vi "Complex Combined System.vi"() -> ()   [LabVIEW 2017]
uses:
  <vilib>/userdefined/High Color/IMAQdx.ctl
  <vilib>/vision/driver/NI_Vision_Acquisition_Software.lvlib
  <vilib>/vision/NI_Vision_Development_Module.lvlib
panel:
  out "String":string
  in  "Send":bool
  out "error out":errorcluster
  out "size(s)":i32
  out "All Other IP Addresses":string
  out "Primary IP Address":string
  in  "Message":string
  in  "Subject":string
  in  "Recipients":string="chyslop@hotmail.co.uk, b8026896@my.shu.ac.uk,"
  in  "Noise IR Sensor 0 = no noise":dbl
  out "Output voltage":dbl
  in  "IR Object Distance":dbl(slide) min=0.0 max=100.0 step=1.0 scale=0.0..0.45
  out "Right Motor Speedometer (m/s)":dbl(knob) scale=-2.5..2.5
  out "Left Motor Speedometer (m/s)":dbl(knob) scale=-2.5..2.5
  in  "Noise Line sesnor 0 = no noise":dbl
  out "Right voltage more than 0?":bool
  out "Right Line sensor output voltage":dbl
  in  "Right Line Detector Sensor":dbl(slide) scale=0.0..5.0
  out "Left Voltage more than 0?":bool
  out "Left Line sensor output voltage":dbl
  in  "Left Line Detector Sensor":dbl(slide) scale=0.0..5.0
  out "Middle voltage more than 0?":bool
  out "Middle Line sensor output voltage":dbl
  in  "Middle Line Detector Sensor":dbl(slide) scale=0.0..5.0
  in  "% Power":dbl(slide) scale=0.0..100.0
  out "Direction":string
  out "Speedometer (m/s)":dbl(knob) scale=0.0..3.0
  out "error out 2":errorcluster
  out "Video Stream":T1(plugin-control)
  in  "stop":bool
  out "Found":bool
  out "Data":string
  out "error out 3":errorcluster
  out "error out 8":errorcluster
  out "error out 4":errorcluster
  in  "Barcode Types To Search":u32[](array[ring])=[6, 4] items=["Reserved", "Codabar", "Code 39", "Code 93", "Code 128", "EAN 8", "EAN 13", "Interleaved 2 of 5", "MSI", "UPCA", "Pharmacode", "RSS Limited"]
  out "error out 5":errorcluster
  in  "Select Vision System":string(combo)="None"
  in  "Session In":T2
  in  "Stop":bool
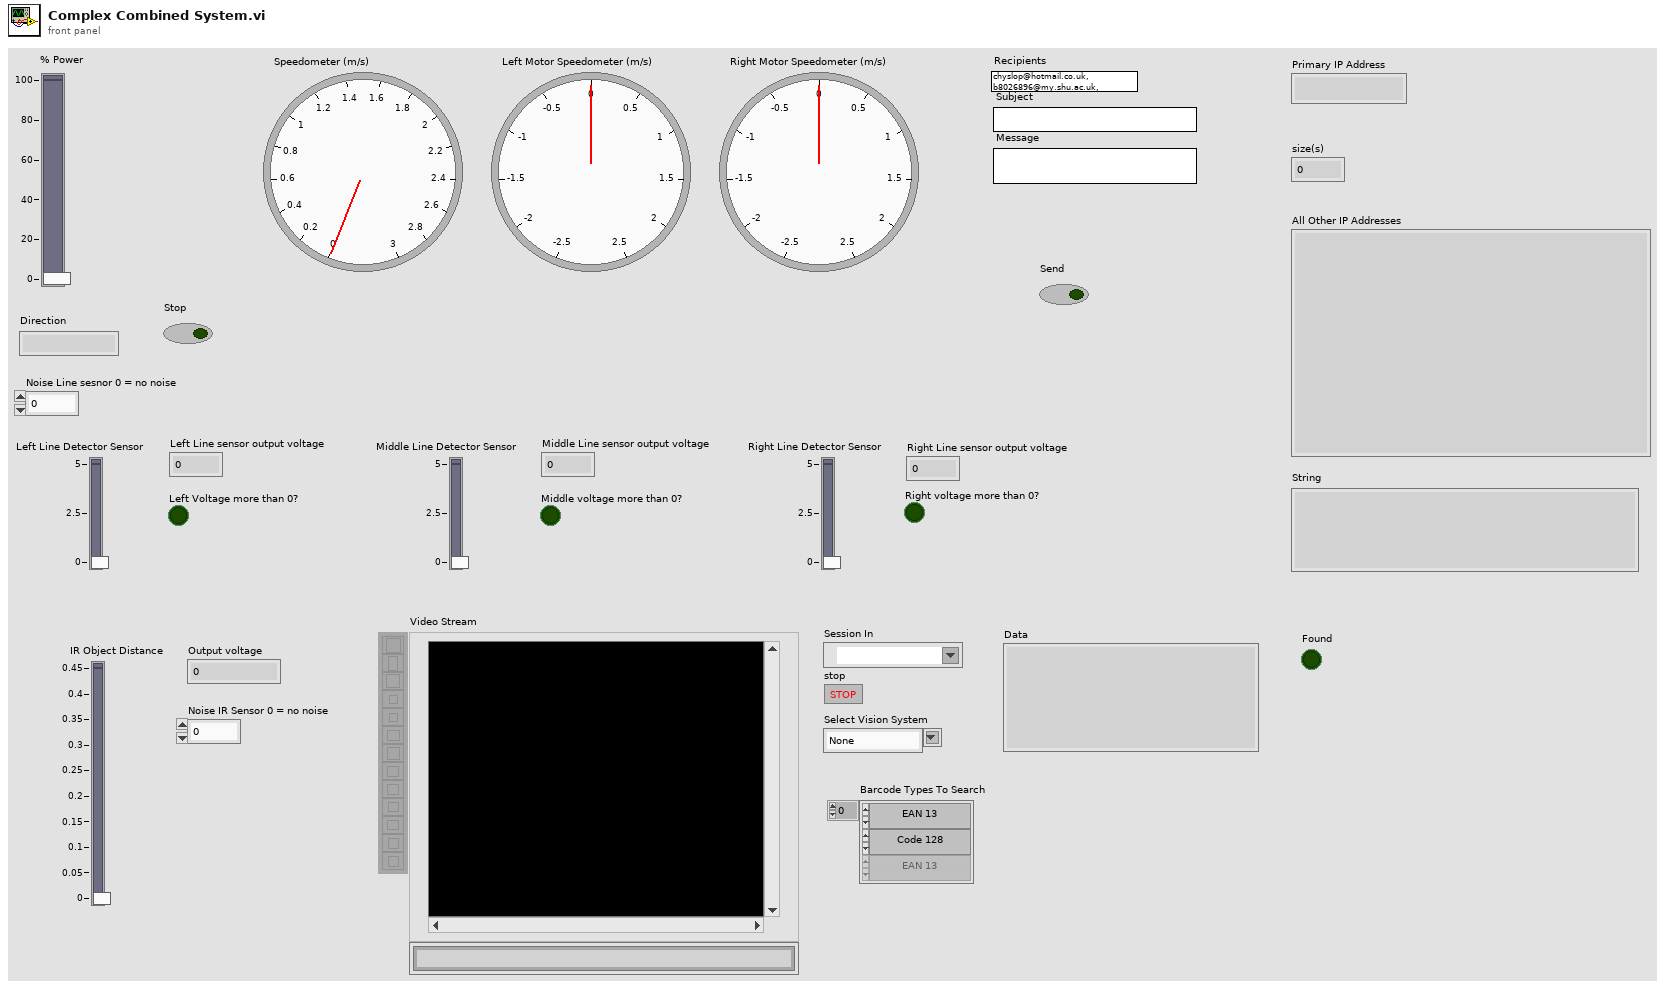
[diagram p1: front panel]
types:
  T1 = typedef "IMAQ Image.ctl" = refnum<image>
  T2 = typedef "IMAQdx.ctl" = refnum<k21>
  T3 = typedef "Image Type" = u32
  T4 = cluster{"Data":string, "Special Char 1":string, "Special Char 2":string, "Checksum(s)":string, "Barcode Type":u32, "Confidence Level":sgl, "Bounding Box":cluster{"x":sgl, "y":sgl}[]}[]
  T5 = cluster{"Data":string, "Special Char 1":string, "Special Char 2":string, "Checksum(s)":string, "Barcode Type":u32, "Confidence Level":sgl, "Bounding Box":cluster{"x":sgl, "y":sgl}[]}
  T6 = typedef "QR Code Report.ctl" = cluster{"Found?":bool, "Data":string, "Bounding Box":cluster{"x":sgl, "y":sgl}[], "Errors Corrected":u32, "Dimensions (Rows/Cols)":u32, "Version":u32, "QR Model":T7, "Stream Mode":T8, "Barcode Polarity":T9, "Mirrored?":bool, "Append Stream Position":u32, "Size of Append Stream":u32, "First EAN-128 ID":i32, "First Alternate Language ID":i32, "Append Stream ID":u32, "Minimum Edge Strength":u32, "Demodulation Mode":T10, "Cell Sample Size":T11, "Cell Filter Mode":T12}
  T7 = typedef "QR Code Model Type.ctl" = i32
  T8 = typedef "QR Code Stream Mode Type.ctl" = i32
  T9 = typedef "Data Matrix Polarity.ctl" = i32
  T10 = typedef "Demodulation Mode.ctl" = i32
  T11 = typedef "Cell Sample Size.ctl" = i32
  T12 = typedef "Cell Filter Mode.ctl" = i32
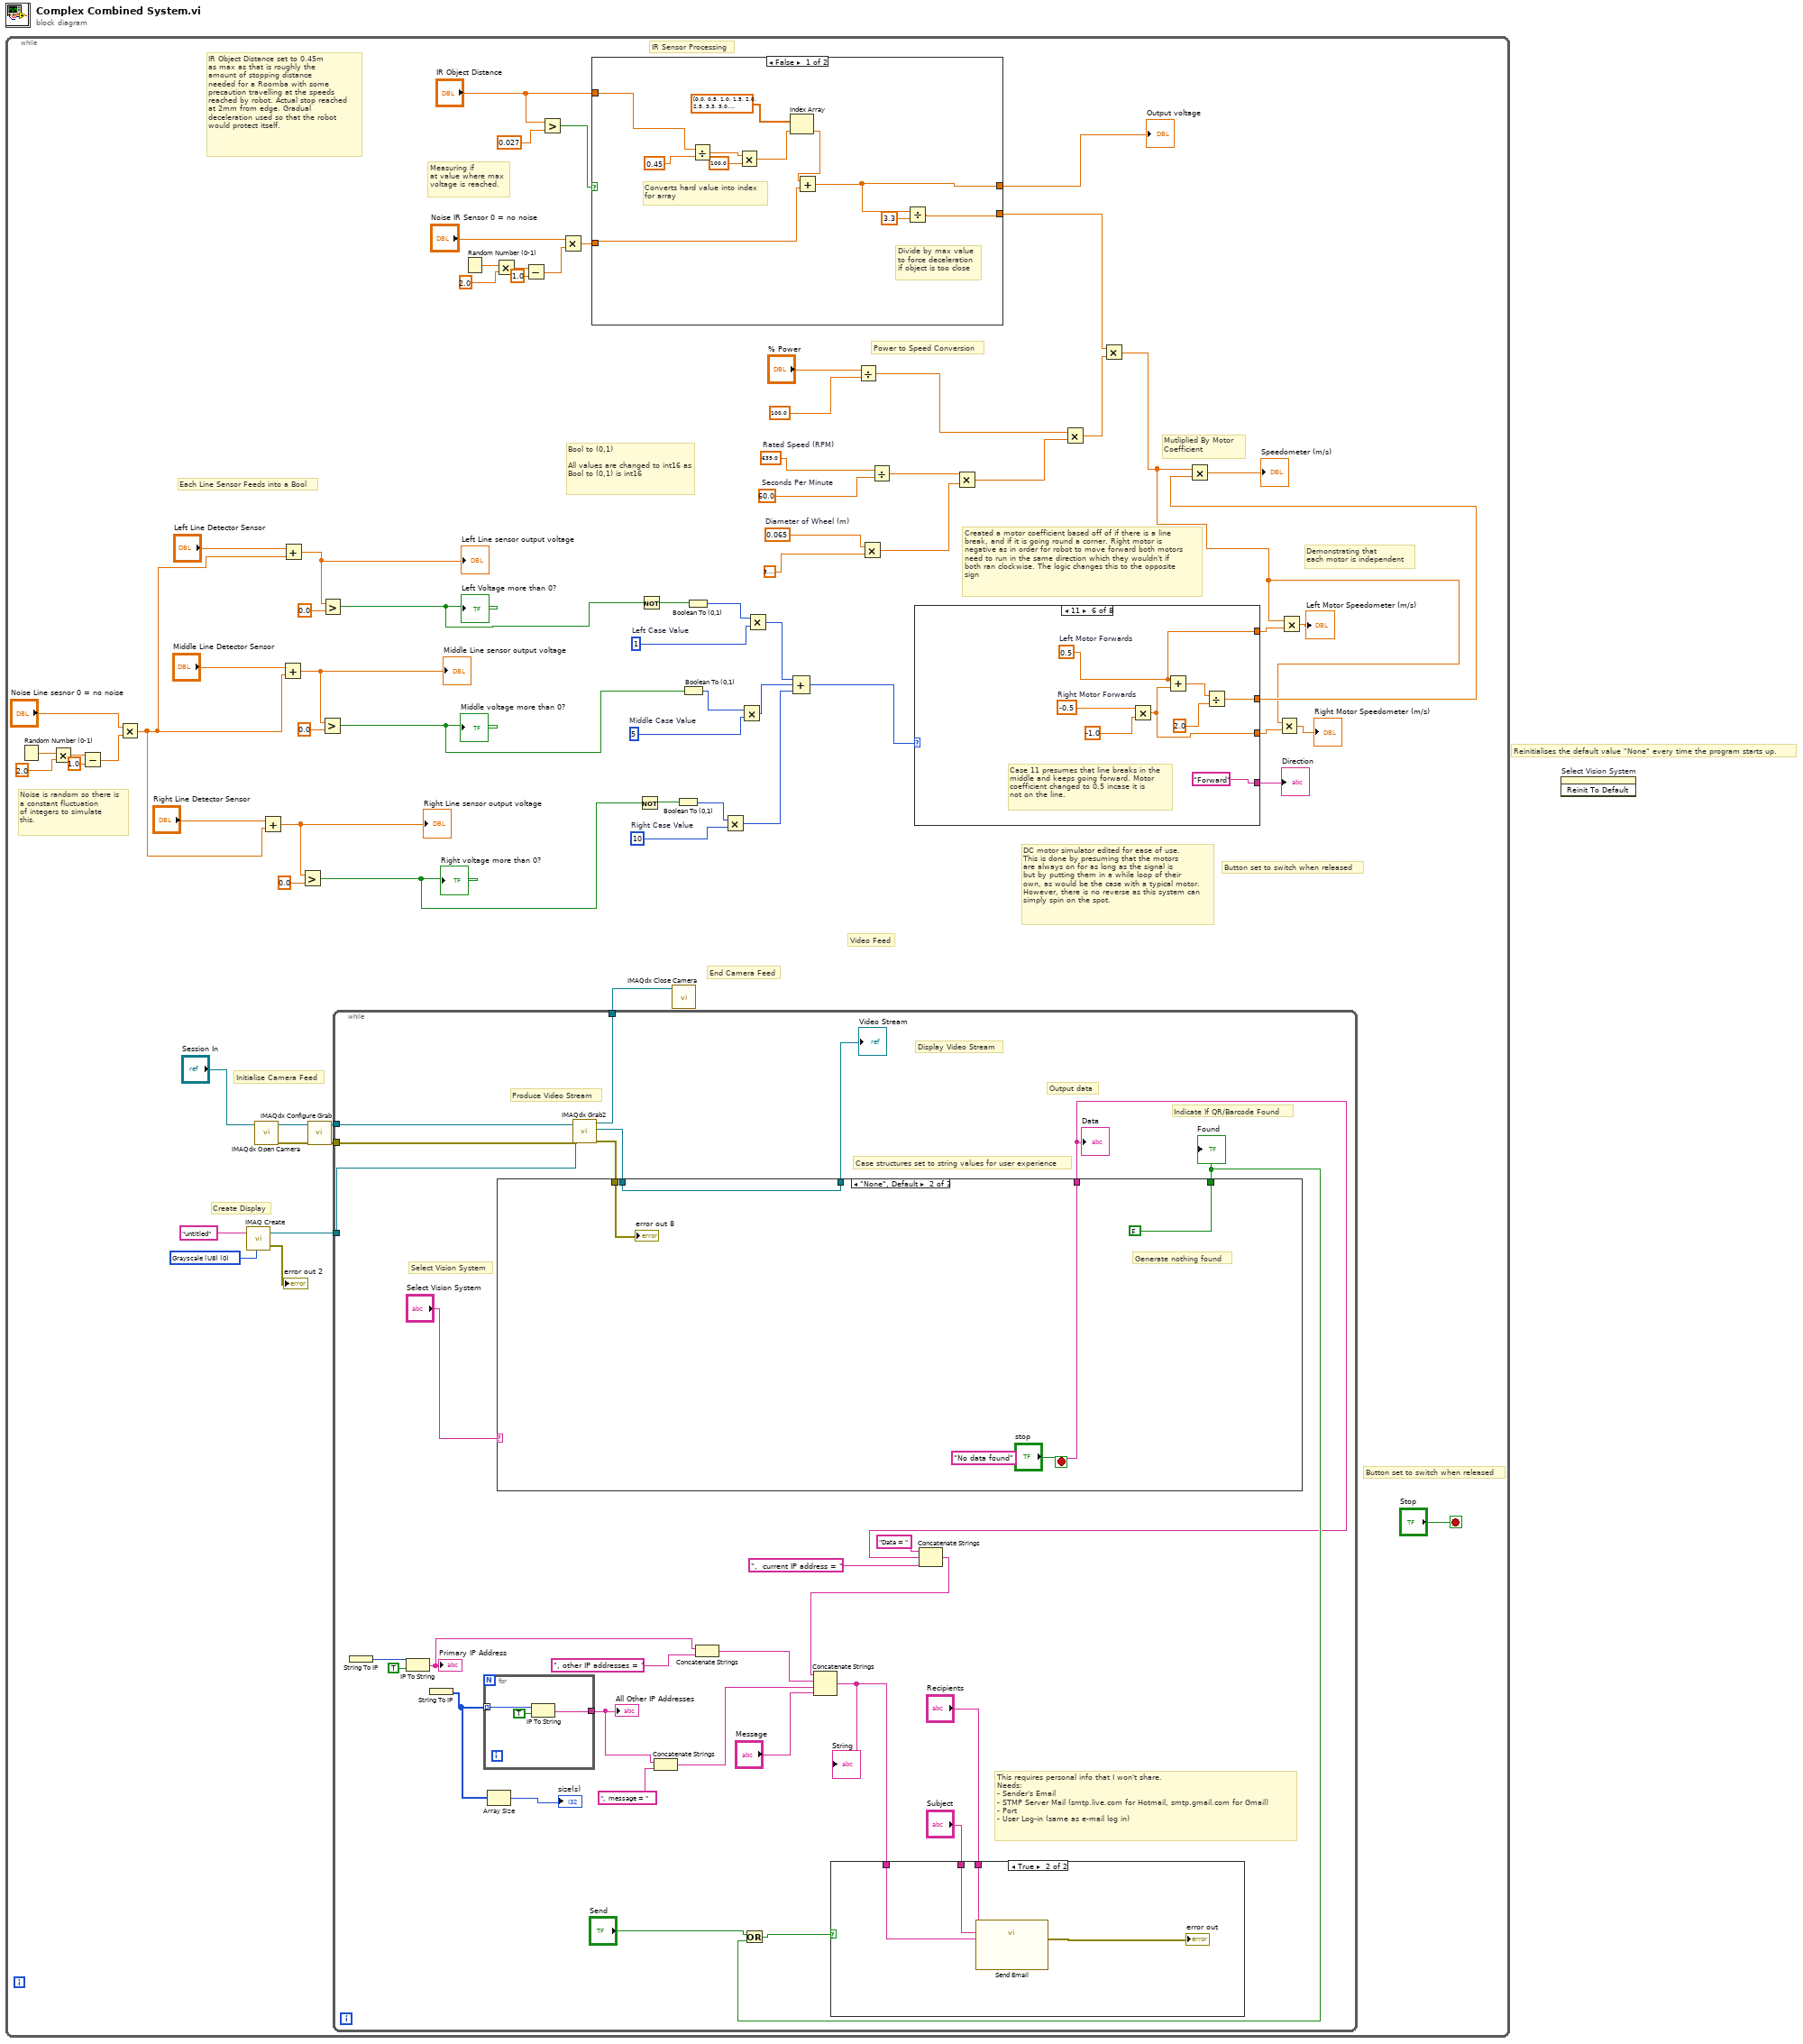
[diagram p0: block diagram]
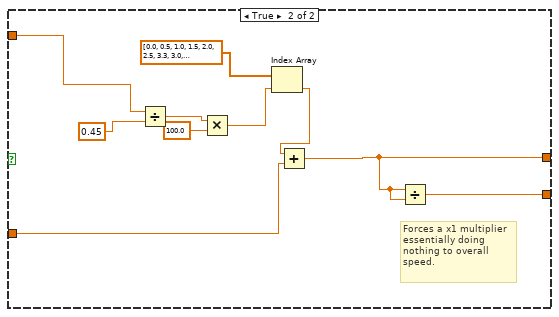
[diagram p2: hidden frame]
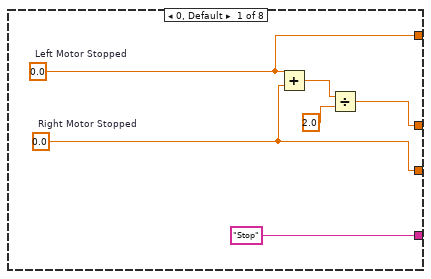
[diagram p3: hidden frame]
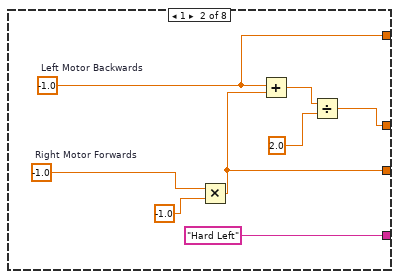
[diagram p4: hidden frame]
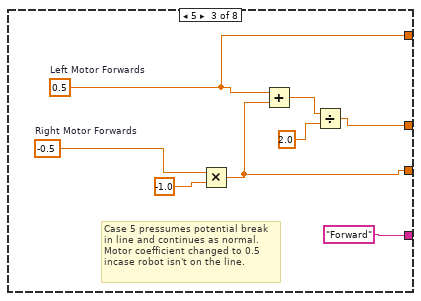
[diagram p5: hidden frame]
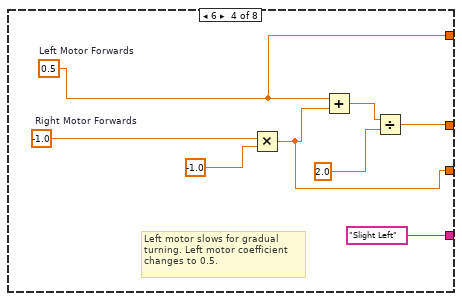
[diagram p6: hidden frame]
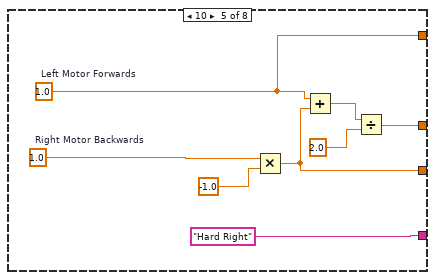
[diagram p7: hidden frame]
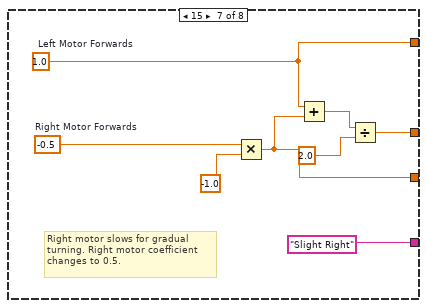
[diagram p8: hidden frame]
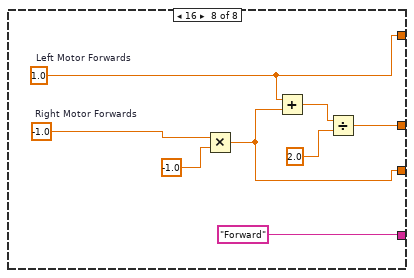
[diagram p9: hidden frame]
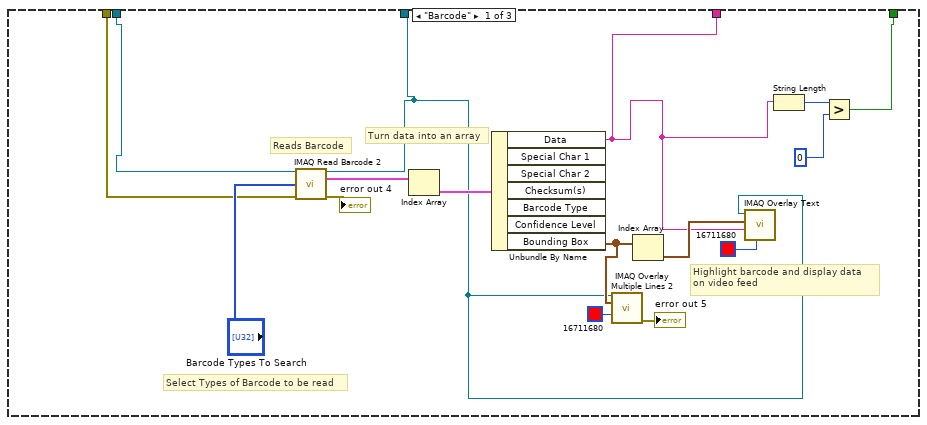
[diagram p11: hidden frame]
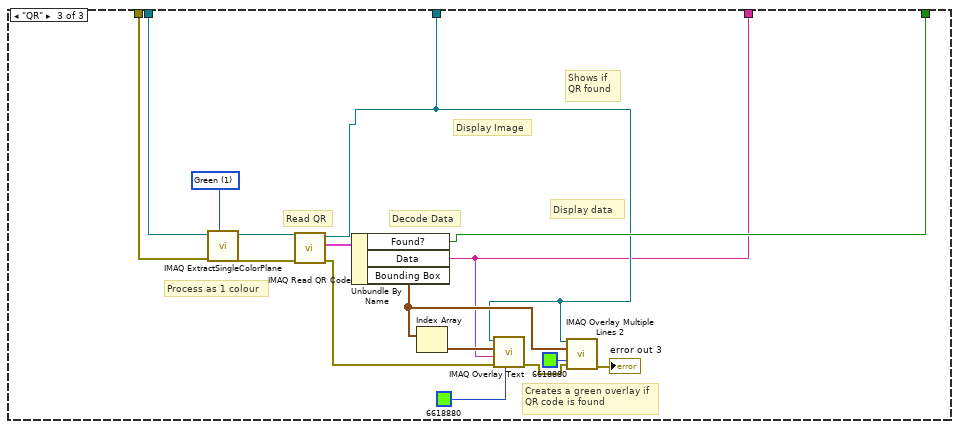
[diagram p12: hidden frame]
diagram:
  # "Reinitialises the default value \"None\" every time the program starts up."
  n1 = while {
    stop <- "Stop" stop-if-true
    w45 = i16 5  # Middle Case Value
    w41 = i16 10  # Right Case Value
    w44 = i16 1  # Left Case Value
    w59 = 0.065  # Diameter of Wheel (m)
    w60 = 60.0  # Seconds Per Minute
    w61 = 639.0  # Rated Speed (RPM)
    w64 = T3 0 items=["Grayscale (U8)", "Grayscale (I16)", "Grayscale (SGL)", "Complex (CSG)", "RGB (U32)", "HSL (U32)", "RGB (U64)", "Grayscale (U16)"] ("Image Type")
    # "IR Object Distance set to 0.45m\nas max as that is roughly the\namount of stopping distance\nneeded for a Roomba with some\nprecaution travelling at the speeds\nreached by robot. Actual stop reached\nat 2mm from edge. Gradual\ndeceleration used so that the robot\nwould protect itself."
    # "Measuring if\nat value where max\nvoltage is reached."
    # "IR Sensor Processing"
    # "Demonstrating that\neach motor is independent"
    # "DC motor simulator edited for ease of use.\nThis is done by presuming that the motors\nare always on for as long as the signal is\nbut by putting them in a while loop of their\nown, as would be the case with a typical motor.\nHowever, there is no reverse as this system can\nsimply spin on the spot."
    # "Noise is random so there is\na constant fluctuation\nof integers to simulate\nthis."
    # "Each Line Sensor Feeds into a Bool"
    # "Created a motor coefficient based off of if there is a line\nbreak, and if it is going round a corner. Right motor is\nnegative as in order for robot to move forward both motors\nneed to run in the same direction which they wouldn't if\nboth ran clockwise. The logic changes this to the opposite\nsign"
    # "Mutliplied By Motor\nCoefficient"
    # "Button set to switch when released"
    # "Bool to (0,1)\n\nAll values are changed to int16 as Bool to (0,1) is int16"
    # "Power to Speed Conversion"
    # "Video Feed"
    # "End Camera Feed"
    # "Create Display"
    # "Initialise Camera Feed"
    # "Button set to switch when released"
    n2 = Random Number (0-1)() -> (number: 0 to 1=w24:dbl)
    n3 = Multiply(x=w24, y=2.0) -> (x*y=w23:dbl)
    n4 = Subtract(x=w23, y=1.0) -> (x-y=w22:dbl)
    n5 = Multiply(x="Noise Line sesnor 0 = no noise", y=w22) -> (x*y=w19:dbl)
    n6 = call "IMAQ Create"("Image Name"="untitled", "Image Type"=w64) -> ("New Image"=w65:T1, "error out"=→"error out 2":errorcluster)  [unwired: 3 in]
    n7 = call <vilib>:"IMAQdx Open Camera.vi"("Session In"="Session In") -> ("error out"=w71:errorcluster, "Session Out"=w72:T2)  [unwired: 9 in]
    n8 = Add(x="Right Line Detector Sensor", y=w19) -> (x+y=w30:dbl)
    "Right Line sensor output voltage" <- w30
    n9 = Add(x="Middle Line Detector Sensor", y=w19) -> (x+y=w36:dbl)
    "Middle Line sensor output voltage" <- w36
    n10 = Add(x="Left Line Detector Sensor", y=w19) -> (x+y=w33:dbl)
    "Left Line sensor output voltage" <- w33
    n11 = Greater?(x=w30, y=0.0) -> (0:w26:bool)
    "Right voltage more than 0?" <- w26
    n12 = call <vilib>:"IMAQdx Configure Grab.vi"("error in"=w71, "Session In"=w72) -> ("error out"=w66:errorcluster, "Session Out"=w68:T2)  [unwired: 8 in]
    n13 = Greater?(x=w36, y=0.0) -> (0:w27:bool)
    "Middle voltage more than 0?" <- w27
    n14 = Greater?(x=w33, y=0.0) -> (0:w28:bool)
    "Left Voltage more than 0?" <- w28
    n15 = while {
      tunnel: w68 -> [w186]
      tunnel: [w185] -> w67
      tunnel: w66 -> [w184]
      tunnel: w65 -> [w183]
      stop <- "stop" stop-if-true
      # "This requires personal info that I won't share.\nNeeds:\n- Sender's Email\n- STMP Server Mail (smtp.live.com for Hotmail, smtp.gmail.com for Gmail)\n- Port\n- User Log-in (same as e-mail log in)"
      # "Output data"
      # "Case structures set to string values for user experience"
      # "Select Vision System"
      # "Indicate If QR/Barcode Found"
      # "Display Video Stream"
      # "Produce Video Stream"
      n16 = String To IP() -> (0:w177:u32)  [unwired: 1 in]
      n17 = IP To String(1:TRUE ("dot notation? (F)"), 2:w177) -> (0:w164:string)
      "Primary IP Address" <- w164
      n18 = String To IP() -> (0:w176:u32[])  [unwired: 1 in]
      n19 = for {
        tunnel: w176 -> [w193] mode=indexing
        tunnel: [w191] -> w160
        n20 = IP To String(1:TRUE ("dot notation? (F)"), 2:w193) -> (0:w191:string)
      }
      "All Other IP Addresses" <- w160
      n21 = Array Size(array=w176) -> (size(s)=→"size(s)":i32)
      n22 = call <vilib>:"IMAQdx Grab2.vi"("error in"=w184, "Image In"=w183, "Session In"=w186) -> ("error out"=w178:errorcluster, "Image Out"=w181:T1, "Session Out"=w185:T2)  [unwired: 5 in, 1 out]
      n23 = case shown="\"None\", Default" "Select Vision System" {
        tunnel: w181 -> [w197 w212 w216]
        tunnel: w178 -> [w196 w213 w215]
        tunnel: [w195 FALSE w218] -> w167
        tunnel: [w198 w212 w217] -> w180
        tunnel: [w194 "No data found" w214] -> w158
        frame "Barcode" {
          # "Highlight barcode and display data\non video feed"
          # "Turn data into an array"
          # "Select Types of Barcode to be read"
          # "Reads Barcode"
          n24 = call "IMAQ Read Barcode 2"("Image"=w197, "Barcode Types To Search"="Barcode Types To Search", "error in (no error)"=w196) -> ("Image (duplicate)"=w198:T1, "Barcodes"=w204:T4, "error out"=→"error out 4":errorcluster)  [unwired: 8 in, 2 out]
          n25 = Index Array(array=w204) -> (element=w205:T5)  [unwired: 1 in]
          n26 = Unbundle By Name(w205) -> ("Data"=w194:string, "Bounding Box"=w207:cluster{"x":sgl, "y":sgl}[])  [unwired: 5 out]
          n27 = call "IMAQ Overlay Multiple Lines 2"("Image"=w198, "Line End Points"=w207, "Color"=u32 16711680) -> ("error out"=→"error out 5":errorcluster)  [unwired: 11 in, 1 out]
          n28 = Index Array(array=w207) -> (element=w206:cluster{"x":sgl, "y":sgl})  [unwired: 1 in]
          n29 = call "IMAQ Overlay Text"("Text Color (black)"=u32 16711680, "String"=w194, "Origin"=w206, "Image"=w198) -> ()  [unwired: 6 in, 2 out]
          n30 = String Length(string=w194) -> (length=w209:i32)
          n31 = Greater?(x=w209, y=0) -> (0:w195:bool)
        }
        frame "None", Default {
          # "Generate nothing found"
          "error out 8" <- w213
        }
        frame "QR" {
          w227 = 1 items=["Red", "Green", "Blue", "Hue", "Saturation", "Luminance", "Value", "Intensity"] ("Color Plane")
          # "Creates a green overlay if\nQR code is found"
          # "Shows if\nQR found"
          # "Display data"
          # "Decode Data"
          # "Display Image"
          # "Read QR"
          # "Process as 1 colour"
          n32 = call "IMAQ ExtractSingleColorPlane"("Color Plane"=w227, "error in (no error)"=w215, "Image Src"=w216) -> ("error out"=w228:errorcluster, "Image Dst Out"=w229:T1)  [unwired: 7 in]
          n33 = call "IMAQ Read QR Code"("error in (no error)"=w228, "Image"=w229) -> ("error out"=w219:errorcluster, "QR Code Report"=w226:T6, "Image (duplicate)"=w217:T1)  [unwired: 6 in, 1 out]
          n34 = Unbundle By Name(w226) -> ("Found?"=w218:bool, "Data"=w214:string, "Bounding Box"=w223:cluster{"x":sgl, "y":sgl}[])
          n35 = Index Array(array=w223) -> (element=w225:cluster{"x":sgl, "y":sgl})  [unwired: 1 in]
          n36 = call "IMAQ Overlay Text"("Text Color (black)"=u32 6618880, "error in (no error)"=w219, "String"=w214, "Origin"=w225, "Image"=w217) -> ("error out"=w221:errorcluster)  [unwired: 5 in, 1 out]
          n37 = call "IMAQ Overlay Multiple Lines 2"("Image"=w217, "Line End Points"=w223, "Color"=u32 6618880, "error in (no error)"=w221) -> ("error out"=→"error out 3":errorcluster)  [unwired: 10 in, 1 out]
        }
      }
      "Video Stream" <- w180
      "Found" <- w167
      "Data" <- w158
      n38 = Concatenate Strings(w160, ",  message = " ("string")) -> (w161:string)
      n39 = Concatenate Strings(w164, ", other IP addresses = " ("string")) -> (w163:string)
      n40 = Or(x="Send", y=w167) -> (x .or. y?=w173:bool)
      n41 = Concatenate Strings("Data = " ("string"), w158, ",  current IP address = " ("string")) -> (w166:string)
      n42 = Concatenate Strings(w166, w163, w161, "Message") -> (w168:string)
      "String" <- w168
      n43 = case shown="True" w173 {
        tunnel: "Subject" -> [_ w189]
        tunnel: "Recipients" -> [_ w188]
        tunnel: w168 -> [_ w187]
        frame False {
        }
        frame True {
          n44 = call "Send Email"("Message"=w187, "Subject"=w189, "Recipients"=w188) -> ("error out"=→"error out":errorcluster)  [unwired: 8 in]
        }
      }
    }
    n45 = Random Number (0-1)() -> (number: 0 to 1=w6:dbl)
    n46 = Multiply(x=w6, y=2.0) -> (x*y=w7:dbl)
    n47 = Subtract(x=w7, y=1.0) -> (x-y=w8:dbl)
    n48 = Greater?(x="IR Object Distance", y=0.027) -> (0:w2:bool)
    n49 = Multiply(x="Noise IR Sensor 0 = no noise", y=w8) -> (x*y=w3:dbl)
    n50 = case shown="False" w2 {
      tunnel: "IR Object Distance" -> [w78 w94]
      tunnel: [w75 w87] -> w14
      tunnel: [w76 w86] -> w1
      tunnel: w3 -> [w77 w85]
      frame False {
        # "Converts hard value into index\nfor array"
        # "Divide by max value\nto force deceleration\nif object is too close"
        n51 = Divide(x=w78, y=0.45) -> (x/y=w83:dbl)
        n52 = Multiply(x=w83, y=100.0) -> (x*y=w84:dbl)
        n53 = Index Array(array=dbl[] [0.0, 0.5, 1.0, 1.5, 2.0, 2.5, 3.3, 3.0, 2.658255897, 2.408413052, 2.20488628, 2.035631323, 1.892484412, 1.769708211, 1.663148013, 1.569718295, 1.487077661, 1.413415986, 1.347310939, 1.287628787, 1.233454287, 1.184040141, 1.138769924, 1.097130449, 1.058690886, 1.023086768, 0.990007602, 0.959187169, 0.930395851, 0.903434503, 0.878129533, 0.854328896, 0.83189883, 0.81072117, 0.790691122, 0.771715412, 0.753710732, 0.736602435, 0.72032343, 0.704813241, 0.690017209, 0.675885801, 0.66237402, 0.64944089, 0.63704902, 0.625164212, 0.613755126, 0.602792986, 0.592251321, 0.582105738, 0.572333717, 0.562914438, 0.553828618, 0.545058374, 0.536587096, 0.528399334, 0.520480698, 0.51281777, 0.50539802, 0.498209735, 0.491241951, 0.484484395, 0.477927433, 0.471562015, 0.465379637, 0.459372298, 0.453532462, 0.447853023, 0.442327281, 0.436948907, 0.431711917, 0.426610656, 0.421639765, 0.416794173, 0.412069067, 0.407459883, 0.402962289, 0.398572167, 0.394285602, 0.39009887, 0.386008427, 0.382010895, 0.378103055, 0.374281838, 0.370544314, 0.366887686, 0.363309281, 0.359806547, 0.35637704, 0.353018422, 0.349728457, 0.346505002, 0.343346003, 0.340249491, 0.337213578, 0.334236453, 0.331316376, 0.328451676, 0.325640748, 0.32288205, 0.320174098] ("first row"), index=w84) -> (element=w82:dbl)
        n54 = Add(x=w82, y=w77) -> (x+y=w75:dbl)
        n55 = Divide(x=w75, y=3.3) -> (x/y=w76:dbl)
      }
      frame True {
        # "Forces a x1 multiplier\nessentially doing\nnothing to overall\nspeed."
        n56 = Divide(x=w94, y=0.45) -> (x/y=w92:dbl)
        n57 = Multiply(x=w92, y=100.0) -> (x*y=w93:dbl)
        n58 = Index Array(array=dbl[] [0.0, 0.5, 1.0, 1.5, 2.0, 2.5, 3.3, 3.0, 2.658255897, 2.408413052, 2.20488628, 2.035631323, 1.892484412, 1.769708211, 1.663148013, 1.569718295, 1.487077661, 1.413415986, 1.347310939, 1.287628787, 1.233454287, 1.184040141, 1.138769924, 1.097130449, 1.058690886, 1.023086768, 0.990007602, 0.959187169, 0.930395851, 0.903434503, 0.878129533, 0.854328896, 0.83189883, 0.81072117, 0.790691122, 0.771715412, 0.753710732, 0.736602435, 0.72032343, 0.704813241, 0.690017209, 0.675885801, 0.66237402, 0.64944089, 0.63704902, 0.625164212, 0.613755126, 0.602792986, 0.592251321, 0.582105738, 0.572333717, 0.562914438, 0.553828618, 0.545058374, 0.536587096, 0.528399334, 0.520480698, 0.51281777, 0.50539802, 0.498209735, 0.491241951, 0.484484395, 0.477927433, 0.471562015, 0.465379637, 0.459372298, 0.453532462, 0.447853023, 0.442327281, 0.436948907, 0.431711917, 0.426610656, 0.421639765, 0.416794173, 0.412069067, 0.407459883, 0.402962289, 0.398572167, 0.394285602, 0.39009887, 0.386008427, 0.382010895, 0.378103055, 0.374281838, 0.370544314, 0.366887686, 0.363309281, 0.359806547, 0.35637704, 0.353018422, 0.349728457, 0.346505002, 0.343346003, 0.340249491, 0.337213578, 0.334236453, 0.331316376, 0.328451676, 0.325640748, 0.32288205, 0.320174098] ("first row"), index=w93) -> (element=w91:dbl)
        n59 = Add(x=w91, y=w85) -> (x+y=w87:dbl)
        n60 = Divide(x=w87, y=w87) -> (x/y=w86:dbl)
      }
    }
    "Output voltage" <- w14
    n61 = Not(x=w26) -> (.not. x?=w38:bool)
    n62 = Not(x=w28) -> (.not. x?=w39:bool)
    n63 = call <vilib>:"IMAQdx Close Camera.vi"("Session In"=w67) -> ()  [unwired: 10 in, 1 out]
    n64 = Boolean To (0,1)(Boolean=w38) -> (0, 1=w49:i16)
    n65 = Boolean To (0,1)(Boolean=w27) -> (0, 1=w46:i16)
    n66 = Boolean To (0,1)(Boolean=w39) -> (0, 1=w50:i16)
    n67 = Multiply(x=w49, y=w41) -> (x*y=w48:i16)
    n68 = Multiply(x=w46, y=w45) -> (x*y=w47:i16)
    n69 = Multiply(x=w50, y=w44) -> (x*y=w51:i16)
    n70 = Compound Arithmetic op=ADD(w51, w47, w48) -> (w43:i16)
    n71 = Divide(x="% Power", y=100.0) -> (x/y=w52:dbl)
    n72 = Multiply(x=w59, y=3.141592653589793) -> (x*y=w56:dbl)
    n73 = Divide(x=w61, y=w60) -> (x/y=w57:dbl)
    n74 = case shown="11" w43 {
      tunnel: ["Stop" "Hard Left" "Forward" "Slight Left" "Hard Right" "Forward" "Slight Right" "Forward"] -> w62
      tunnel: [w97 w105 w113 w121 w129 w137 w145 w153] -> w40
      tunnel: [w95 w102 w109 w117 w126 w133 w141 w150] -> w16
      tunnel: [w96 w101 w110 w118 w125 w134 w142 w149] -> w18
      frame 0, Default {
        w95 = 0.0  # Right Motor Stopped
        w96 = 0.0  # Left Motor Stopped
        n75 = Add(x=w96, y=w95) -> (x+y=w99:dbl)
        n76 = Divide(x=w99, y=2.0) -> (x/y=w97:dbl)
      }
      frame 1 {
        w103 = -1.0  # Right Motor Forwards
        w101 = -1.0  # Left Motor Backwards
        n77 = Multiply(x=w103, y=-1.0) -> (x*y=w102:dbl)
        n78 = Add(x=w101, y=w102) -> (x+y=w107:dbl)
        n79 = Divide(x=w107, y=2.0) -> (x/y=w105:dbl)
      }
      frame 5 {
        w111 = -0.5  # Right Motor Forwards
        w110 = 0.5  # Left Motor Forwards
        # "Case 5 pressumes potential break\nin line and continues as normal.\nMotor coefficient changed to 0.5\nincase robot isn't on the line."
        n80 = Multiply(x=w111, y=-1.0) -> (x*y=w109:dbl)
        n81 = Add(x=w110, y=w109) -> (x+y=w115:dbl)
        n82 = Divide(x=w115, y=2.0) -> (x/y=w113:dbl)
      }
      frame 6 {
        w119 = -1.0  # Right Motor Forwards
        w118 = 0.5  # Left Motor Forwards
        # "Left motor slows for gradual\nturning. Left motor coefficient\nchanges to 0.5."
        n83 = Multiply(x=w119, y=-1.0) -> (x*y=w117:dbl)
        n84 = Add(x=w118, y=w117) -> (x+y=w123:dbl)
        n85 = Divide(x=w123, y=2.0) -> (x/y=w121:dbl)
      }
      frame 10 {
        w127 = 1.0  # Right Motor Backwards
        w125 = 1.0  # Left Motor Forwards
        n86 = Multiply(x=w127, y=-1.0) -> (x*y=w126:dbl)
        n87 = Add(x=w125, y=w126) -> (x+y=w131:dbl)
        n88 = Divide(x=w131, y=2.0) -> (x/y=w129:dbl)
      }
      frame 11 {
        w135 = -0.5  # Right Motor Forwards
        w134 = 0.5  # Left Motor Forwards
        # "Case 11 presumes that line breaks in the \nmiddle and keeps going forward. Motor\ncoefficient changed to 0.5 incase it is\nnot on the line."
        n89 = Multiply(x=w135, y=-1.0) -> (x*y=w133:dbl)
        n90 = Add(x=w134, y=w133) -> (x+y=w139:dbl)
        n91 = Divide(x=w139, y=2.0) -> (x/y=w137:dbl)
      }
      frame 15 {
        w143 = -0.5  # Right Motor Forwards
        w142 = 1.0  # Left Motor Forwards
        # "Right motor slows for gradual\nturning. Right motor coefficient\nchanges to 0.5."
        n92 = Multiply(x=w143, y=-1.0) -> (x*y=w141:dbl)
        n93 = Add(x=w142, y=w141) -> (x+y=w147:dbl)
        n94 = Divide(x=w147, y=2.0) -> (x/y=w145:dbl)
      }
      frame 16 {
        w151 = -1.0  # Right Motor Forwards
        w149 = 1.0  # Left Motor Forwards
        n95 = Multiply(x=w151, y=-1.0) -> (x*y=w150:dbl)
        n96 = Add(x=w149, y=w150) -> (x+y=w155:dbl)
        n97 = Divide(x=w155, y=2.0) -> (x/y=w153:dbl)
      }
    }
    "Direction" <- w62
    n98 = Multiply(x=w57, y=w56) -> (x*y=w55:dbl)
    n99 = Multiply(x=w52, y=w55) -> (x*y=w10:dbl)
    n100 = Multiply(x=w1, y=w10) -> (x*y=w9:dbl)
    n101 = Multiply(x=w9, y=w40) -> (x*y=→"Speedometer (m/s)":dbl)
    n102 = Multiply(x=w9, y=w16) -> (x*y=→"Right Motor Speedometer (m/s)":dbl)
    n103 = Multiply(x=w9, y=w18) -> (x*y=→"Left Motor Speedometer (m/s)":dbl)
  }
  n104 = invoke on="Select Vision System" class="CmbBox" method="Reinit To Default"() -> ()  [unwired: 3 in, 3 out]
